vi "DTC.ValueCode.Set.vi"(8 "error in":errorcluster, 11 "Section Ref in":T1 format="%.0x") -> (0 "error out":errorcluster, 3 "Section Ref out":T1 format="%.0x")   [LabVIEW 2019, in "Diagnostics Addon System Explorer.lvlib"]
uses:
  Diagnostics Addon System Explorer.lvlib
  <vilib>/NI VeriStand/Custom Device Tools/Custom Device Utility Library/Custom Device Utility Library.lvlib
  Shared/SubVIs/Constants.vi
  Shared/Diagnostics Addon Shared.lvlib
  <vilib>/NI VeriStand/Custom Device API/Custom Device API.lvlib
  Types/FG.Action.ctl
  <vilib>/NI VeriStand/Custom Device Tools/Custom Device Utility Library/NI VeriStand - Search for Item by Name.vi
  <vilib>/NI VeriStand/Custom Device Tools/Custom Device Utility Library/NI VeriStand - Search for All Items by GUID.vi
  <vilib>/NI VeriStand/Custom Device API/Custom Device Item Ref.ctl
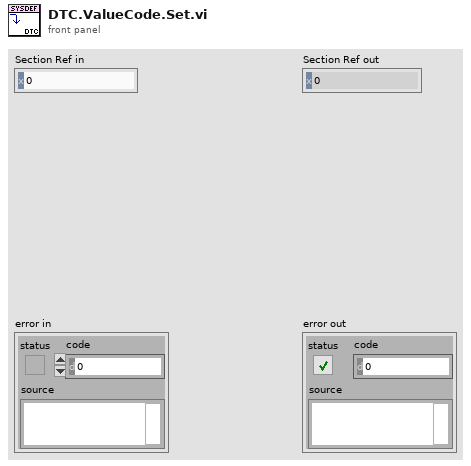
[diagram p1: front panel]
types:
  T1 = typedef "Custom Device API.lvlib/Custom Device Item Ref.ctl" = u64
  T2 = typedef "Diagnostics Addon System Explorer.lvlib/FG.Action.ctl" = enum16{"Get", "Set"}
  T3 = typedef "Diagnostics Addon Shared.lvlib/DTC.Settings.ctl" = cluster{"Descriptor":T4, "Value.Code":dbl[], "Value.String":string[], "Value.J2012String":string[], "Status.Code":dbl[], "Status.String":string[]}
  T4 = typedef "Diagnostics Addon Shared.lvlib/DTC.Descriptor.ctl" = cluster{"DTC Byte Length":i32, "Status Byte Length":i32, "Add Data Byte Length":i32, "Byte Order":enum16{"Motorola", "Intel"}}
  T5 = typedef "Custom Device API.lvlib/Custom Device Item Info.ctl" = cluster{"Name":string, "Is Channel":bool, "GUID":string, "Is Waveform":bool}
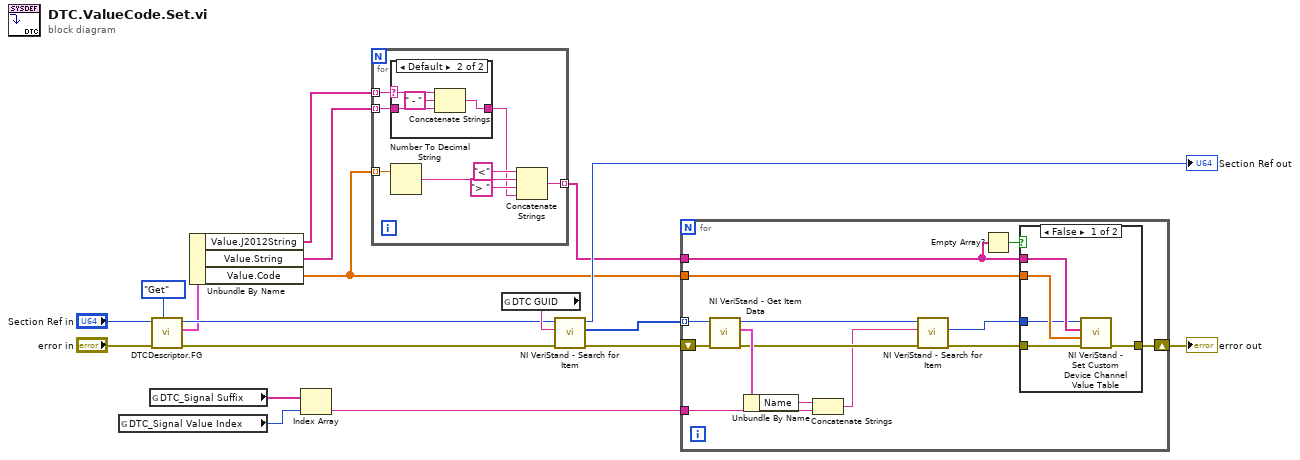
[diagram p0: block diagram]
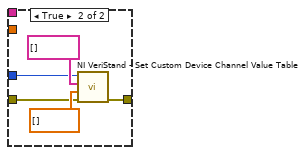
[diagram p3: hidden frame]
diagram:
  n1 = global read "Constants.vi" "DTC_Signal Value Index"() -> (w16:i32)
  n2 = global read "Constants.vi" "DTC_Signal Suffix"() -> (w17:string[])
  n3 = call "DTCDescriptor.FG.vi"("Action"=FG.Action."Get", "error in (no error)"="error in", "Device Item Ref in"="Section Ref in") -> ("error out"=w8:errorcluster, "DTC descriptor"=w5:T3, "Device Item Ref out"=w6:T1)  [unwired: 6 in]
  n4 = Unbundle By Name(w5) -> ("Value.J2012String"=w4:string[], "Value.String"=w3:string[], "Value.Code"=w1:dbl[])
  n5 = Index Array(array=w17, index=w16) -> (element=w13:string)
  n6 = for {
    tunnel: w3 -> [w26] mode=indexing
    tunnel: w4 -> [w25] mode=indexing
    tunnel: [w19] -> w2 mode=indexing
    tunnel: w1 -> [w24] mode=indexing
    n7 = case shown="Default" w25 {
      selector: w25 -> [_ w29]
      tunnel: w26 -> [w27 w30]
      tunnel: [w27 w28] -> w20
      frame "" {
      }
      frame Default {
        n8 = Concatenate Strings(w29, " - " ("string"), w30) -> (w28:string)
      }
    }
    n9 = Number To Decimal String(number=w24) -> (decimal integer string=w21:string)  [unwired: 1 in]
    n10 = Concatenate Strings("<" ("string"), w21, "> " ("string"), w20) -> (w19:string)
  }
  n11 = global read "Constants.vi" "DTC GUID"() -> (w18:string)
  n12 = call-poly <vilib>:"NI VeriStand - Search for Item.vi"("error in"=w8, "Item GUID"=w18, "Section Ref in"=w6) -> ("error out"=w15:errorcluster, "Item Refs"=w14:T1[], "Section Ref out"=→"Section Ref out":T1)  [unwired: 5 in, 1 out]
  n13 = for {
    shift-right: [w42] -> w12
    shift-left: w15 -> [w35]
    tunnel: w14 -> [w37] mode=indexing
    tunnel: w13 -> [w33]
    tunnel: w2 -> [w41]
    tunnel: w1 -> [w40]
    n14 = call <vilib>:"NI VeriStand - Get Item Data.vi"("error in (no error)"=w35, "Item Ref in"=w37) -> ("error out"=w34:errorcluster, "Item Info"=w39:T5, "Item Ref out"=w36:T1)  [unwired: 6 in, 1 out]
    n15 = Unbundle By Name(w39) -> ("Name"=w38:string)
    n16 = Concatenate Strings(w38, w33) -> (w32:string)
    n17 = call-poly <vilib>:"NI VeriStand - Search for Item.vi"("error in"=w34, "Item Name"=w32, "Section Ref in"=w36) -> ("error out"=w43:errorcluster, "Item Ref"=w44:T1)  [unwired: 5 in, 2 out]
    n18 = Empty Array?(array=w41) -> (empty?=w45:bool)
    n19 = case shown="False" w45 {
      tunnel: w41 -> [w50 _]
      tunnel: w40 -> [w49 _]
      tunnel: [w48 w55] -> w42
      tunnel: w44 -> [w46 w52]
      tunnel: w43 -> [w47 w51]
      frame False {
        n20 = call <vilib>:"NI VeriStand - Set Custom Device Channel Value Table.vi"("error in (no error)"=w47, "Values"=w49, "Names"=w50, "Channel Ref in"=w46) -> ("error out"=w48:errorcluster)  [unwired: 6 in, 1 out]
      }
      frame True {
        n21 = call <vilib>:"NI VeriStand - Set Custom Device Channel Value Table.vi"("error in (no error)"=w51, "Values"=dbl[] [], "Names"=string[] [], "Channel Ref in"=w52) -> ("error out"=w55:errorcluster)  [unwired: 6 in, 1 out]
      }
    }
  }
  "error out" <- w12
